vi "Actor Core.vi"(8 "error in":errorcluster, 11 "MQTT-Client in":refnum<class "MQTT-Client.lvclass">) -> (0 "error out":errorcluster, 3 "Actor out":refnum<class "Actor.lvclass">)   [LabVIEW 2023, in "MQTT-Client.lvlib" / "MQTT-Client.lvclass"]
doc: "(<B>Filename</B>: Actor Framework.lvlib:Actor.lvclass:Actor Core.vi)\n\nReceives messages to the actor, reacts to them, and initiates any error handling that may shut the actor down.\n\nDescendant classes may override this VI to append parallel tasks for the actor to complete while it handles messages. Overrides use the Call Parent Class Method node."
uses:
  MQTT-Client.lvclass
  <vilib>/ActorFramework/Actor/Actor.lvclass
  CustomFlat/CustomFlat.lvclass
  C:/Program Files/National Instruments/LabVIEW 2023/vi.lib/LabVIEW Open Source Project/OpenSerializer/Serializer/Serializer.lvclass
  MQTT-Client.lvclass/MQTT-Client.ctl
  <vilib>/LabVIEW Open Source Project/MQTT Connection/MQTT_Base/Base Class/MQTT_Base.lvclass/MQTT_Base.ctl
  <vilib>/LabVIEW Open Source Project/MQTT Client/Client class/Client.lvclass/Client.ctl
  Message.ctl
  <vilib>/LabVIEW Open Source Project/Connection/Connection.TCP/Connection.TCP.lvclass
  C:/Program Files/National Instruments/LabVIEW 2023/vi.lib/LabVIEW Open Source Project/Connection/Connection/Connection.lvclass
  <vilib>/LabVIEW Open Source Project/MQTT Client/Client class/Client.lvclass
  C:/Program Files/National Instruments/LabVIEW 2023/vi.lib/LabVIEW Open Source Project/MQTT Connection/MQTT_Base/Base Class/MQTT_Base.lvclass
  <vilib>/LabVIEW Open Source Project/OpenSerializer/Serializer.FlattenedString/Serializer.FlattenedString.lvclass
  <vilib>/LabVIEW Open Source Project/OpenSerializer/Serializer/Serializer.lvclass
  <vilib>/LabVIEW Open Source Project/MQTT Control Packets/Control Packets/PUBLISH/PUBLISH.lvclass
  <vilib>/LabVIEW Open Source Project/MQTT Connection/MQTT_Base/Base Class/MQTT_Base.lvclass
  C:/Program Files/National Instruments/LabVIEW 2023/vi.lib/LabVIEW Open Source Project/MQTT Client/Client class/Client.lvclass
panel:
  out "Chart":dbl(graph)
  in  "Scheduling":i32 min=-1 format="%.0f ms"
  out "Unsuback":bool
  out "Suback":bool
  in  "Subscribe":bool
  in  "Connection":bool
  out "Published":bool
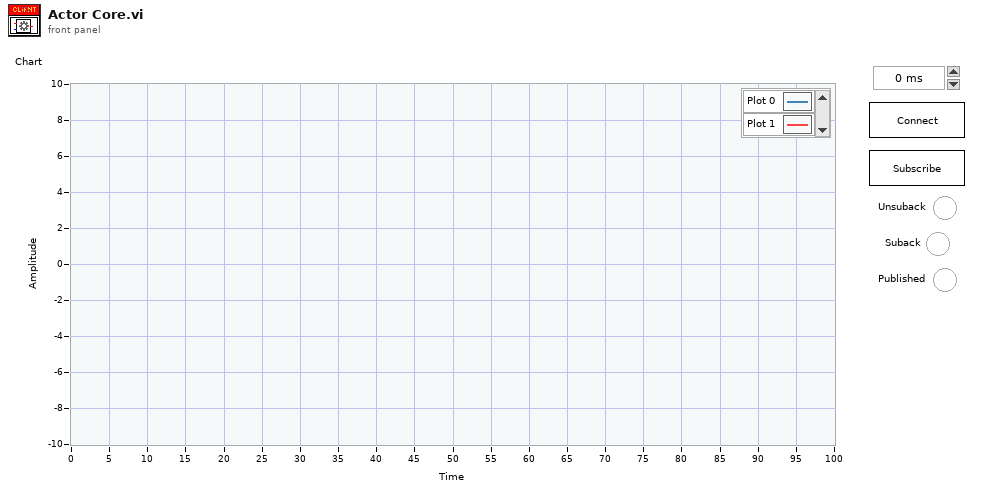
[diagram p1: front panel]
types:
  T1 = typedef "MQTT Client.lvlib/Client.lvclass/Public Events -- cluster.ctl" = cluster{"Connection Status":refnum<user-event>, "Connected":refnum<user-event>, "Application Message":refnum<user-event>}
  T2 = typedef "MQTT Base.lvlib/MQTT_Base.lvclass/Public Events -- cluster.ctl" = cluster{"Stop Event":refnum<user-event>, "Error Event":refnum<user-event>, "Inbound Message":refnum<user-event>}
  T3 = typedef "Message.ctl" = cluster{"Time":dbl, "Payload":string}
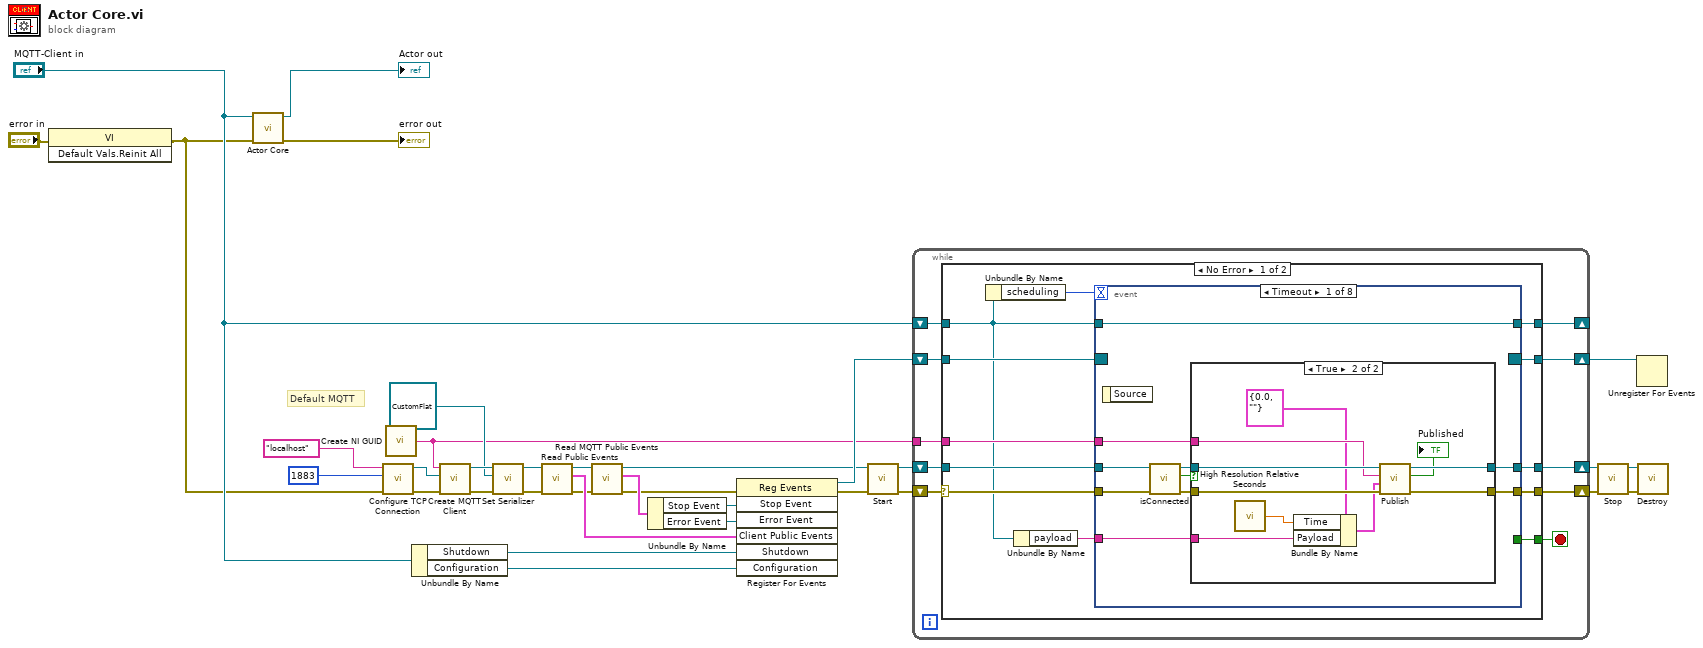
[diagram p0: block diagram]
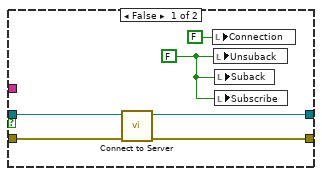
[diagram p2: hidden frame]
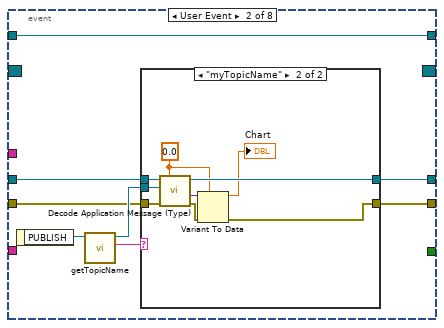
[diagram p3: hidden frame]
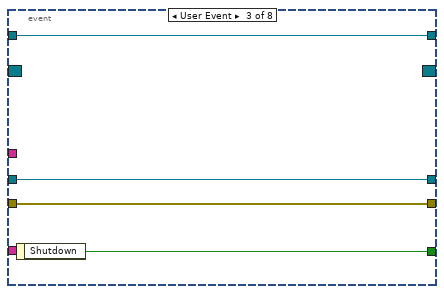
[diagram p5: hidden frame]
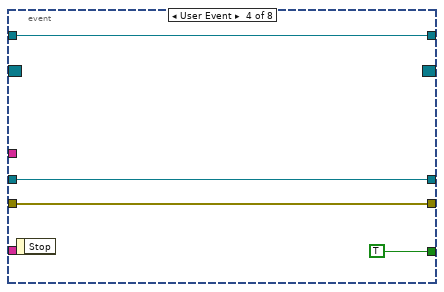
[diagram p6: hidden frame]
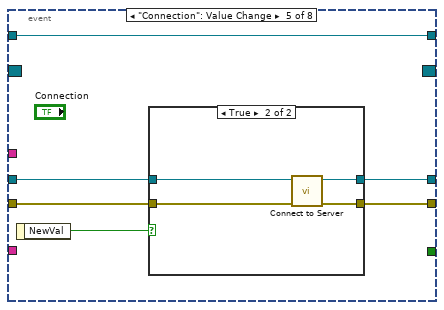
[diagram p7: hidden frame]
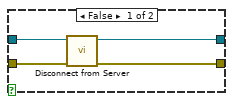
[diagram p8: hidden frame]
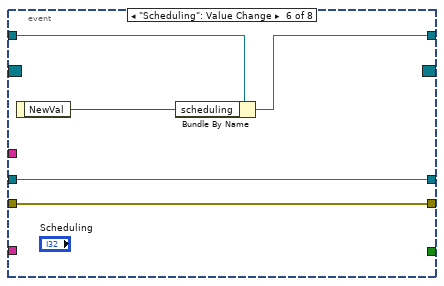
[diagram p9: hidden frame]
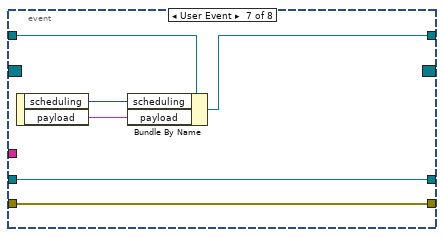
[diagram p10: hidden frame]
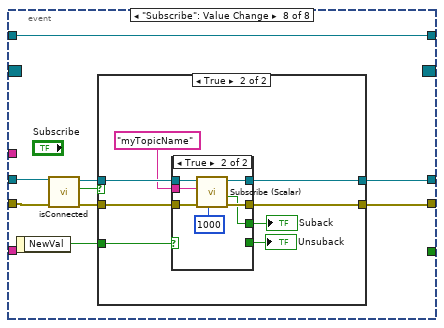
[diagram p11: hidden frame]
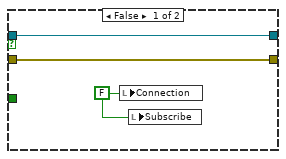
[diagram p12: hidden frame]
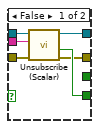
[diagram p13: hidden frame]
diagram:
  # "Default MQTT"
  n1 = invoke class="VI" method="Default Vals.Reinit All"(error in="error in") -> (error out=w1:errorcluster)  [unwired: 2 in, 2 out]
  n2 = call-parent "Actor Core.vi"("error in"=w1, "Actor in"="MQTT-Client in") -> ("error out"=→"error out":errorcluster, "Actor out"=→"Actor out":refnum<class "Actor.lvclass">)  [unwired: 8 in]
  n3 = call <vilib>:"Configure TCP Connection.vi"("error in (no error)"=w1, "remote port (80)"=u16 1883, "address (localhost)"="localhost") -> ("error out"=w12:errorcluster, "Connection.TCP"=w32:refnum<class "Connection.TCP.lvclass">)  [unwired: 7 in]
  n4 = call <vilib>:"Create NI GUID.vi"() -> ("NI GUID"=w5:string)
  n5 = Unbundle By Name("MQTT-Client in") -> ("Shutdown"=w11:refnum<user-event>, "Configuration"=w4:refnum<user-event>)
  n6 = call <vilib>:"Create MQTT Client.vi"("error in (no error)"=w12, "Connection Configuration"=w32, "ID (empty:generate new)"=w5) -> ("error out"=w10:errorcluster, "Client out"=w9:refnum<class "Client.lvclass">)  [unwired: 7 in]
  n7 = call <vilib>:"Set Serializer.vi"("error in (no error)"=w10, "Serializer (default: Flattened String)"=refnum<class "CustomFlat.lvclass"> refnum ("CustomFlat.lvclass"), "MQTT_Base"=w9) -> ("error out"=w7:errorcluster, "MQTT_Base out"=w6:refnum<class "Client.lvclass">)  [unwired: 7 in]
  n8 = call <vilib>:"Read Public Events.vi"("error in (no error)"=w7, "Client in"=w6) -> ("error out"=w16:errorcluster, "Client Public Events"=w18:T1, "Client out"=w15:refnum<class "Client.lvclass">)  [unwired: 7 in]
  n9 = call <vilib>:"Read MQTT Public Events.vi"("error in (no error)"=w16, "MQTT_Base in"=w15) -> ("error out"=w17:errorcluster, "MQTT Public Events"=w25:T2, "MQTT_Base out"=w20:refnum<class "Client.lvclass">)  [unwired: 7 in]
  n10 = Unbundle By Name(w25) -> ("Stop Event"=w23:refnum<user-event>, "Error Event"=w24:refnum<user-event>)
  n11 = register-events(error in=w17, w23, w24, w18, w11, w4) -> (reference out=w21:refnum<event-registration>, error out=w19:errorcluster)  [unwired: 1 in]
  n12 = call <vilib>:"Start.vi"("error in (no error)"=w19, "MQTT_Base in"=w20) -> ("error out"=w31:errorcluster, "MQTT_Base out"=w30:refnum<class "Client.lvclass">)  [unwired: 7 in, 1 out]
  n13 = while {
    shift-right: [w43] -> w22
    shift-left: w21 -> [w44]
    shift-right: [w40] -> w27
    shift-left: w30 -> [w41]
    shift-right: [w42] -> w29
    shift-left: w31 -> [w38]
    tunnel: w5 -> [w37]
    shift-right: [w35] -> _
    shift-left: "MQTT-Client in" -> [w36]
    stop <- w39 stop-if-true
    n14 = case shown="No Error" w38 {
      selector: w38 -> [w50 _]
      tunnel: w44 -> [w56 w168]
      tunnel: [w55 w168] -> w43
      tunnel: [w54 _] -> w42
      tunnel: w41 -> [w53 w169]
      tunnel: [w52 w169] -> w40
      tunnel: [w51 _] -> w39
      tunnel: w37 -> [w49 _]
      tunnel: w36 -> [w46 w170]
      tunnel: [w48 w170] -> w35
      frame No Error {
        n15 = Unbundle By Name(w46) -> ("scheduling"=w47:i32)
        n16 = Unbundle By Name(w46) -> ("payload"=w45:string)
        n17 = event shown="[0] Timeout" {
          selector: w56 -> [_ _ _ _ _ _ _ _]
          dyn-events: [_ _ _ _ _ _ _ _] -> w55
          timeout: w47 -> [_ _ _ _ _ _ _ _]
          tunnel: w50 -> [w62 w87 w104 w109 w111 w128 w134 w141]
          tunnel: [w65 w84 w104 w109 w112 w128 w134 w142] -> w54
          tunnel: [_ _ w103 TRUE _ _ _ _] -> w51
          tunnel: w53 -> [w64 w88 w105 w107 w115 w127 w133 w140]
          tunnel: [w66 w86 w105 w107 w113 w127 w133 w143] -> w52
          tunnel: w49 -> [w59 _ _ _ _ _ _ _]
          tunnel: w46 -> [w58 w83 w102 w106 w110 w126 w130 w135]
          tunnel: [w58 w83 w102 w106 w110 w124 w129 w135] -> w48
          tunnel: w45 -> [w57 _ _ _ _ _ _ _]
          event Timeout {
            n18 = event-data() -> ()  [unwired: 1 in, 1 out]
            n19 = call <vilib>:"isConnected.vi"("error in (no error)"=w62, "Client in"=w64) -> ("error out"=w61:errorcluster, "connected"=w60:bool, "Client out"=w63:refnum<class "Client.lvclass">)  [unwired: 7 in]
            n20 = case shown="True" w60 {
              tunnel: [w67 w81] -> w66
              tunnel: [w68 w79] -> w65
              tunnel: w63 -> [w69 w82]
              tunnel: w61 -> [w70 w80]
              tunnel: w59 -> [_ w77]
              tunnel: w57 -> [_ w73]
              frame False {
                w72 = FALSE
                n21 = call <vilib>:"Connect to Server.vi"("error in (no error)"=w70, "Client in"=w69) -> ("error out"=w68:errorcluster, "Client out"=w67:refnum<class "Client.lvclass">)  [unwired: 6 in, 2 out]
                n22 = local write "Connection"(FALSE ("Connection")) -> ()
                n23 = local write "Unsuback"(w72) -> ()
                n24 = local write "Suback"(w72) -> ()
                n25 = local write "Subscribe"(w72) -> ()
              }
              frame True {
                n26 = call <vilib>:"High Resolution Relative Seconds.vi"() -> ("relative seconds"=w75:dbl)
                n27 = Bundle By Name(cluster=T3 {"Time"=0.0, "Payload"=""} ("Message"), "Time"=w75, "Payload"=w73) -> (w74:T3)
                n28 = call <vilib>:"Publish.vi"("error in (no error)"=w80, "Payload"=w74, "Topic Name (empty: Payload name)"=w77, "Client in"=w82) -> ("error out"=w79:errorcluster, "Published"=→"Published":bool, "Client out"=w81:refnum<class "Client.lvclass">)  [unwired: 5 in]
              }
            }
          }
          event User Event {
            n29 = event-data() -> ("PUBLISH"=w90:refnum<class "PUBLISH.lvclass">)  [unwired: 1 in]
            n30 = call <vilib>:"getTopicName.vi"("PUBLISH in"=w90) -> ("Topic"=w85:string, "PUBLISH out"=w89:refnum<class "PUBLISH.lvclass">)  [unwired: 8 in, 1 out]
            n31 = case shown="\"myTopicName\"" w85 {
              tunnel: w89 -> [_ w99]
              tunnel: w88 -> [w92 w100]
              tunnel: w87 -> [w91 w98]
              tunnel: [w92 w95] -> w86
              tunnel: [w91 w101] -> w84
              frame Default {
              }
              frame "myTopicName" {
                w94 = 0.0
                n32 = call <vilib>:"Decode Application Message (Type).vi"("Type"=w94, "error in (no error)"=w98, "PUBLISH"=w99, "Client in"=w100) -> ("error out"=w97:errorcluster, "Payload"=w96:variant, "Client out"=w95:refnum<class "Client.lvclass">)  [unwired: 4 in, 1 out]
                n33 = Variant To Data(error in=w97, type=w94, Variant=w96) -> (data=→"Chart":dbl, error out=w101:errorcluster)
              }
            }
          }
          event User Event {
            n34 = event-data() -> ("Shutdown"=w103:bool)  [unwired: 1 in]
          }
          event User Event {
            n35 = event-data() -> ()  [unwired: 1 in, 1 out]
          }
          event "Connection": Value Change {
            n36 = event-data() -> ("NewVal"=w114:bool)  [unwired: 1 in]
            n37 = case shown="True" w114 {
              tunnel: w115 -> [w119 w123]
              tunnel: [w118 w120] -> w113
              tunnel: [w117 w121] -> w112
              tunnel: w111 -> [w116 w122]
              frame False {
                n38 = call <vilib>:"Disconnect from Server.vi"("error in (no error)"=w116, "Client in"=w119) -> ("error out"=w117:errorcluster, "Client out"=w118:refnum<class "Client.lvclass">)  [unwired: 7 in, 1 out]
              }
              frame True {
                n39 = call <vilib>:"Connect to Server.vi"("error in (no error)"=w122, "Client in"=w123) -> ("error out"=w121:errorcluster, "Client out"=w120:refnum<class "Client.lvclass">)  [unwired: 6 in, 2 out]
              }
            }
          }
          event "Scheduling": Value Change {
            n40 = event-data() -> ("NewVal"=w125:i32)  [unwired: 1 in]
            n41 = Bundle By Name(cluster=w126, "scheduling"=w125) -> (w124:refnum<class "MQTT-Client.lvclass">)
          }
          event User Event {
            n42 = event-data() -> ("scheduling"=w132:i32, "payload"=w131:string)  [unwired: 1 in]
            n43 = Bundle By Name(cluster=w130, "scheduling"=w132, "payload"=w131) -> (w129:refnum<class "MQTT-Client.lvclass">)
          }
          event "Subscribe": Value Change {
            n44 = event-data() -> ("NewVal"=w136:bool)  [unwired: 1 in]
            n45 = call <vilib>:"isConnected.vi"("error in (no error)"=w141, "Client in"=w140) -> ("error out"=w138:errorcluster, "connected"=w137:bool, "Client out"=w139:refnum<class "Client.lvclass">)  [unwired: 7 in]
            n46 = case shown="True" w137 {
              tunnel: [w146 w154] -> w143
              tunnel: [w145 w153] -> w142
              tunnel: w139 -> [w146 w152]
              tunnel: w138 -> [w145 w151]
              tunnel: w136 -> [_ w149]
              frame False {
                w144 = FALSE ("Connection")
                n47 = local write "Connection"(w144) -> ()
                n48 = local write "Subscribe"(w144) -> ()
              }
              frame True {
                n49 = case shown="True" w149 {
                  tunnel: [w157 w166] -> w154
                  tunnel: [w155 w163] -> w153
                  tunnel: w152 -> [w160 w167]
                  tunnel: w151 -> [w159 w164]
                  tunnel: "myTopicName" ("Topic Name (empty: Payload name)") -> [w158 w165]
                  tunnel: [_ w162] -> w148
                  tunnel: [w156 _] -> w147
                  frame False {
                    n50 = call <vilib>:"Unsubscribe (Scalar).vi"("error in (no error)"=w159, "Topic Filter"=w158, "Client in"=w160) -> ("error out"=w155:errorcluster, "Ack"=w156:bool, "Client out"=w157:refnum<class "Client.lvclass">)  [unwired: 6 in]
                  }
                  frame True {
                    n51 = call <vilib>:"Subscribe (Scalar).vi"("timeout (1000ms)"=1000 ("timeout (100ms)"), "error in (no error)"=w164, "Topic Filter"=w165, "Client in"=w167) -> ("error out"=w163:errorcluster, "Ack"=w162:bool, "Client out"=w166:refnum<class "Client.lvclass">)  [unwired: 5 in]
                  }
                }
                "Unsuback" <- w147
                "Suback" <- w148
              }
            }
          }
        }
      }
      frame Error {
      }
    }
  }
  n52 = call <vilib>:"Stop.vi"("error in (no error)"=w29, "MQTT_Base in"=w27) -> ("error out"=w28:errorcluster, "MQTT_Base out"=w26:refnum<class "Client.lvclass">)  [unwired: 7 in, 1 out]
  n53 = Unregister For Events(event registration refnum=w22) -> ()  [unwired: 1 in, 1 out]
  n54 = call <vilib>:"Destroy.vi"("error in (no error)"=w28, "MQTT_Base in"=w26) -> ()  [unwired: 8 in, 2 out]
